vi "Voltage_vs_field.vi"() -> ()   [LabVIEW 2015]
uses:
  <vilib>/Utility/file.llb/Write To Spreadsheet File (string).vi
panel:
  out "Data Point":i32
  out "PS Output (A)":dbl
  in  "Filename Label (optional)":string
  out "Voltage (uV)":dbl
  out "Field (Oe)":dbl
  in  "Power Supply Precision (2-5)":dbl=3.0
  in  "Save Output to:":path=path "C:/VNA-FMR user/Desktop/HV loop"
  in  "Voltmeter Rate (0.1-5)":string="5"
  in  "Gaussmeter Address":string="22"
  in  "Nano Voltmeter Address":string="9"
  in  "Power Supply Address":string="6"
  out "XY Graph":cluster{dbl[], dbl[]}(graph)
  in  "Data Points":dbl=501.0
  in  "Field Range (Oe)":dbl=500.0
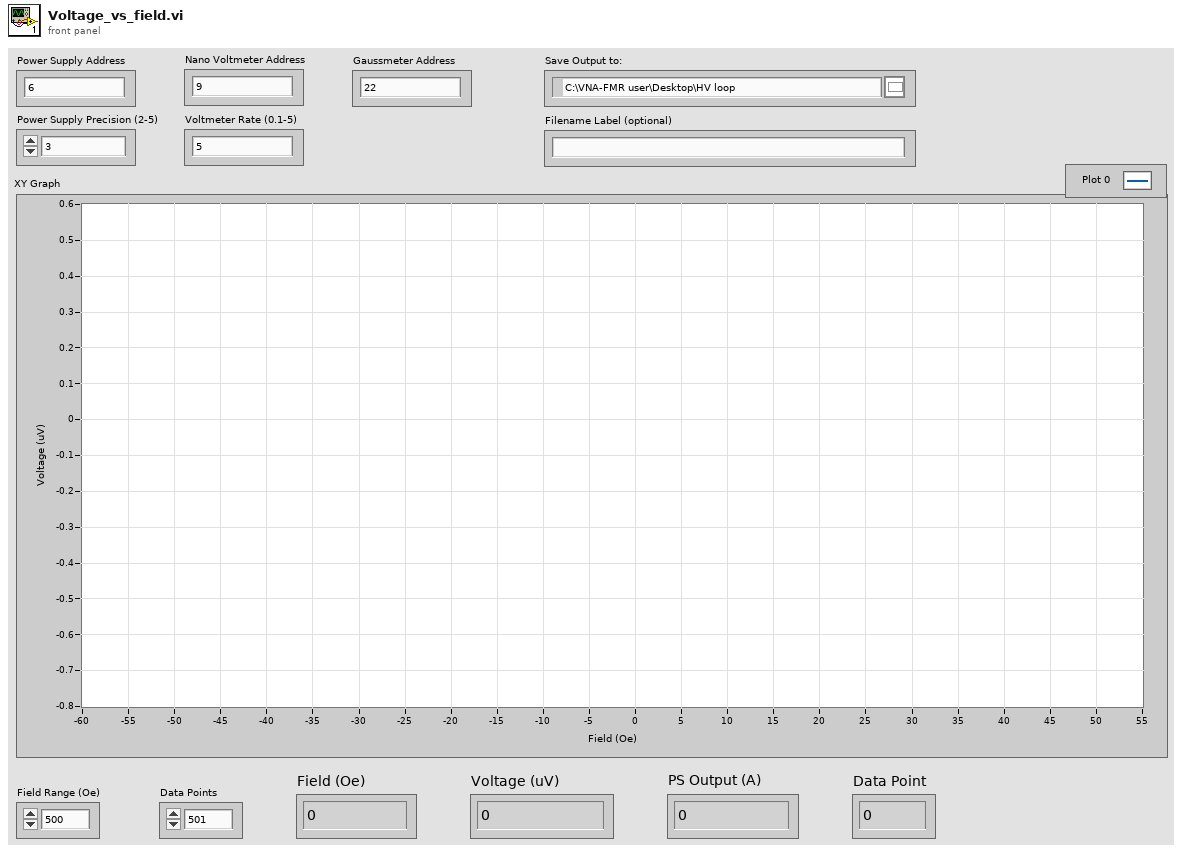
[diagram p1: front panel]
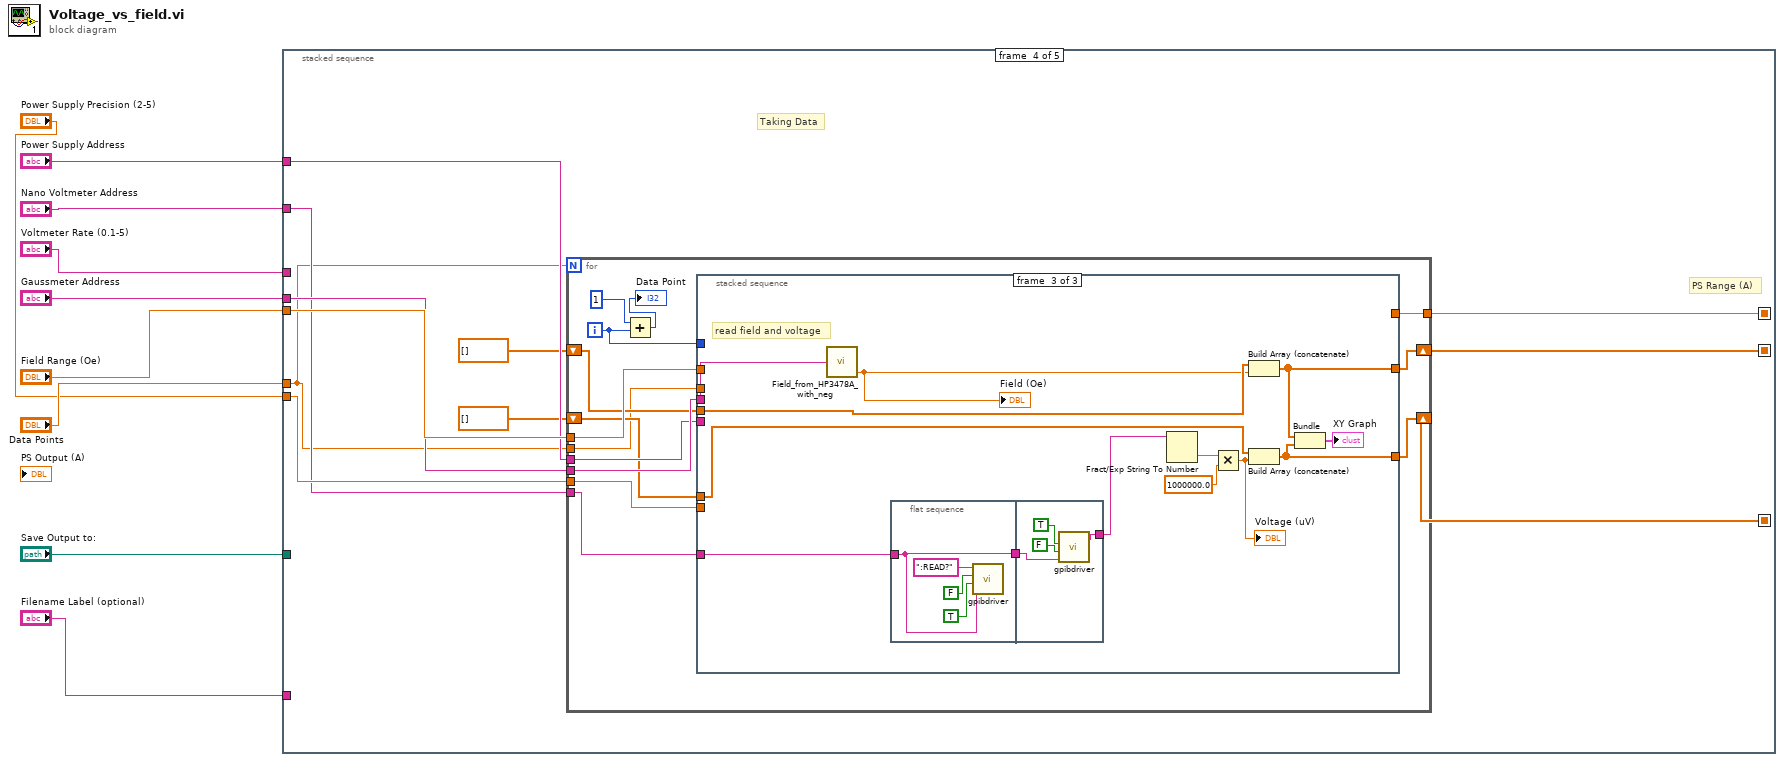
[diagram p0: block diagram]
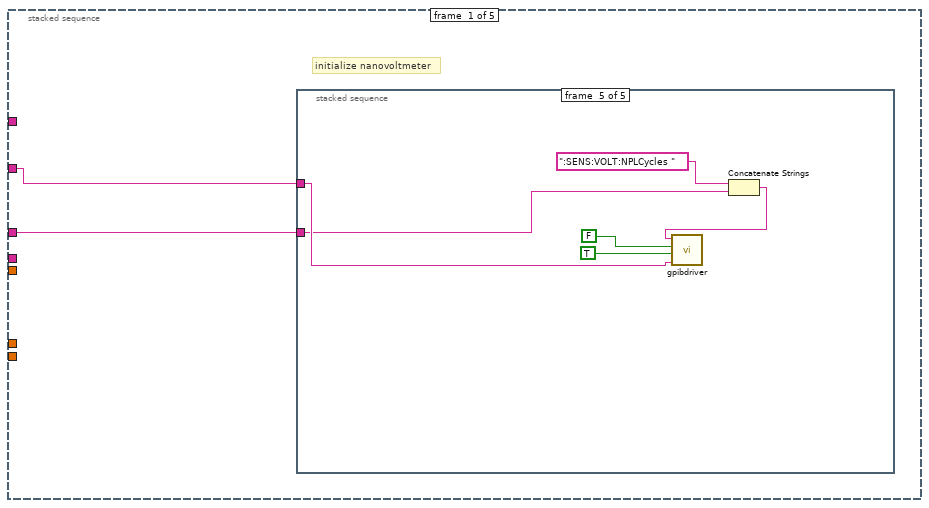
[diagram p2: hidden frame]
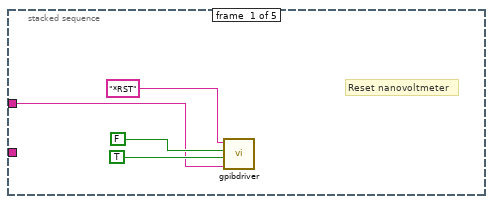
[diagram p3: hidden frame]
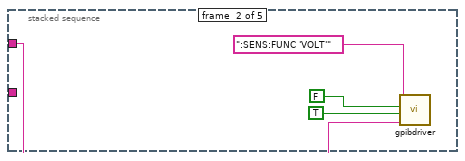
[diagram p4: hidden frame]
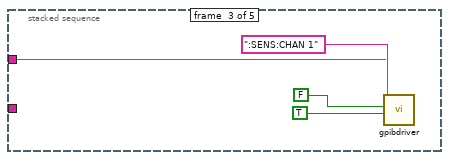
[diagram p5: hidden frame]
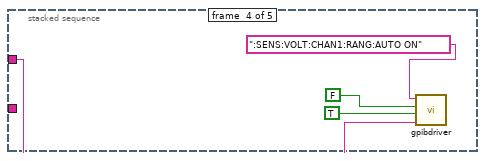
[diagram p6: hidden frame]
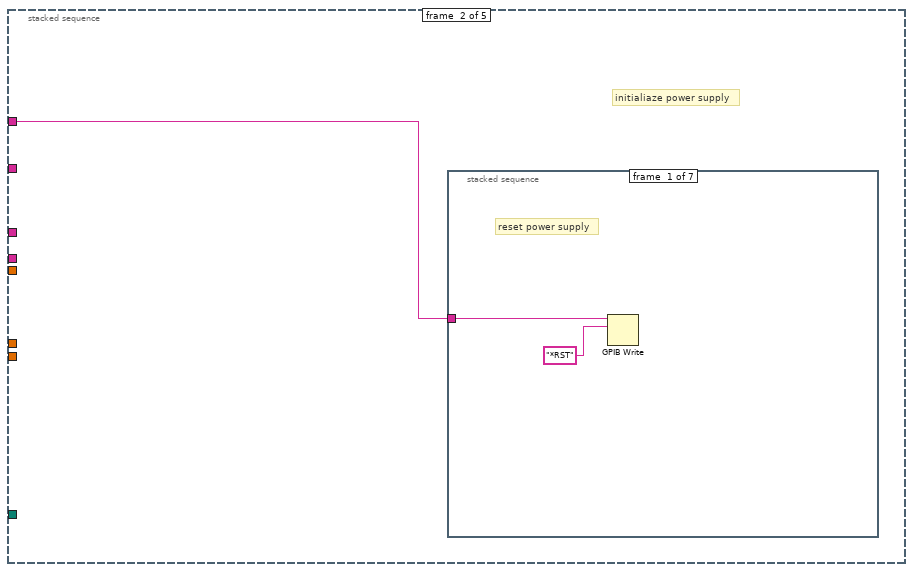
[diagram p7: hidden frame]
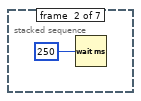
[diagram p8: hidden frame]
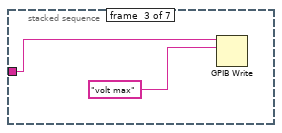
[diagram p9: hidden frame]
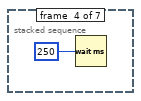
[diagram p10: hidden frame]
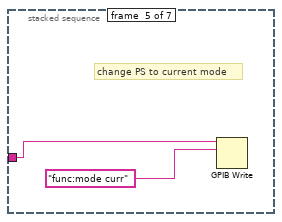
[diagram p11: hidden frame]
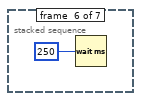
[diagram p12: hidden frame]
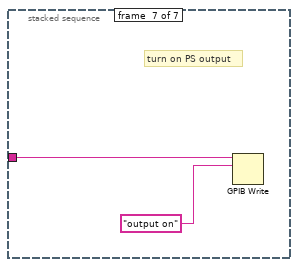
[diagram p13: hidden frame]
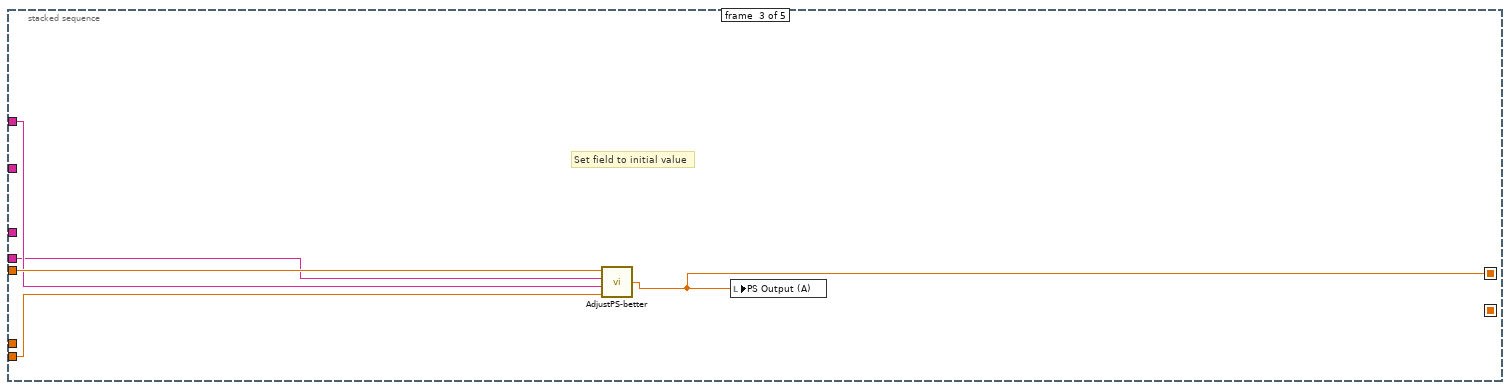
[diagram p14: hidden frame]
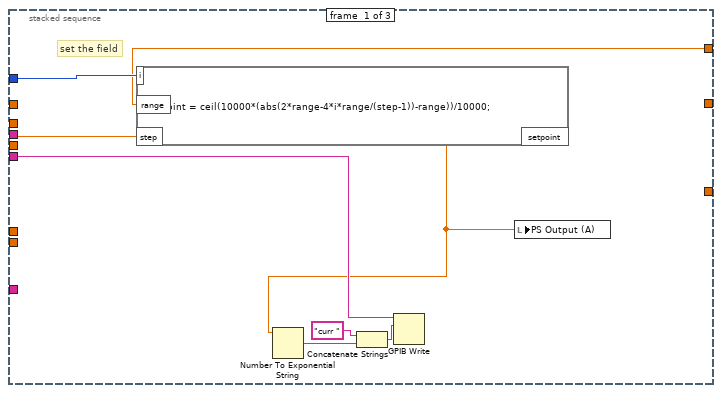
[diagram p15: hidden frame]
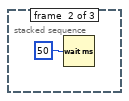
[diagram p16: hidden frame]
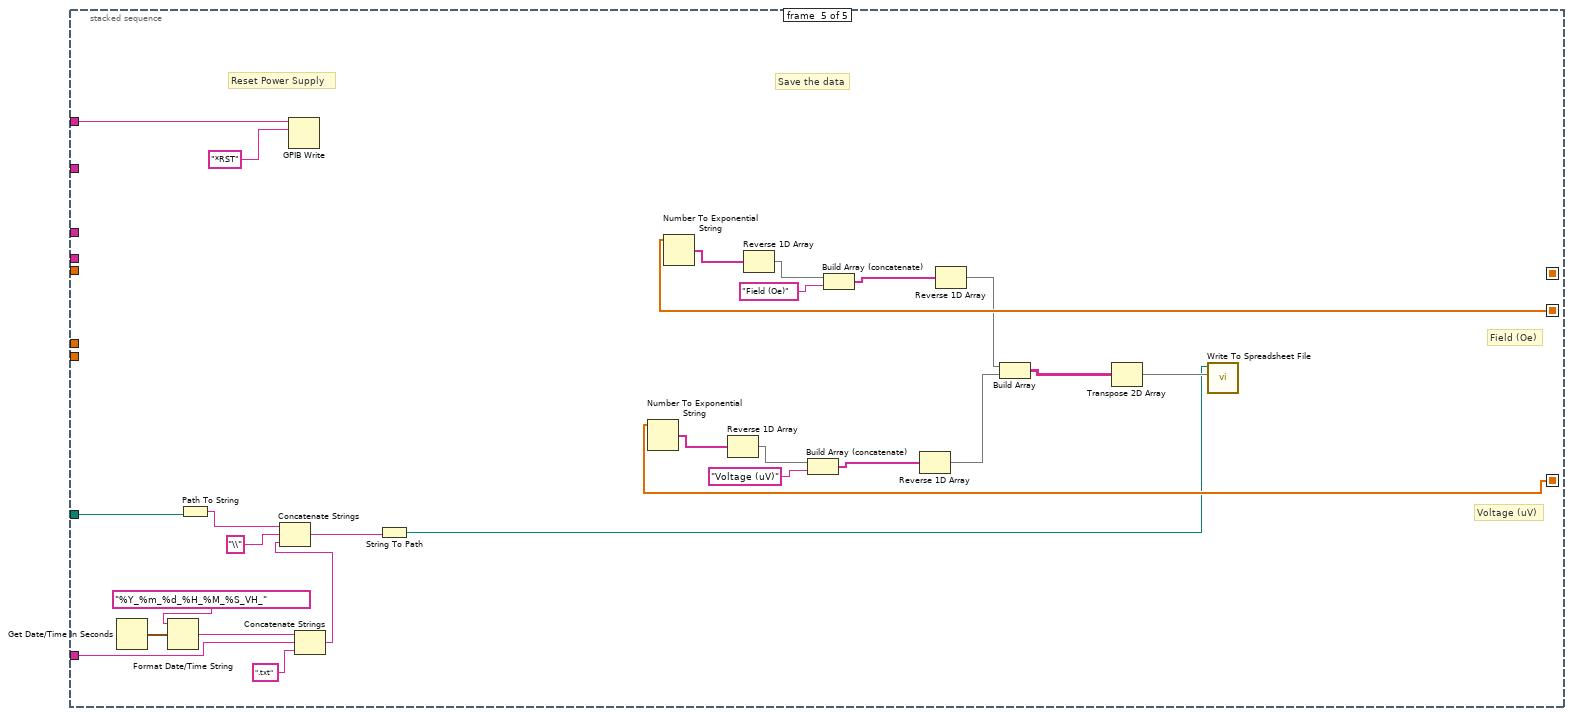
[diagram p17: hidden frame]
diagram:
  n1 = stacked-sequence {
    seq-local: [_ _ _ w54 _] -> [_ _ _ _ w125]
    seq-local: [_ _ _ w53 _] -> [_ _ _ _ w118]
    seq-local: [_ _ w46 _ _] -> [_ _ _ w51 _]
    tunnel: "Nano Voltmeter Address" -> [w11 _ _ w57 _]
    tunnel: "Voltmeter Rate (0.1-5)" -> [w10 _ _ _ _]
    tunnel: "Power Supply Address" -> [_ w34 w49 w59 w132]
    tunnel: "Field Range (Oe)" -> [_ _ w50 w61 _]
    tunnel: "Gaussmeter Address" -> [_ _ w48 w60 _]
    tunnel: "Data Points" -> [_ _ _ w52 _]
    tunnel: "Power Supply Precision (2-5)" -> [_ _ w47 w58 _]
    tunnel: "Save Output to:" -> [_ _ _ _ w116]
    tunnel: "Filename Label (optional)" -> [_ _ _ _ w108]
    frame #0 {
      # "initialize nanovoltmeter"
      n2 = stacked-sequence {
        tunnel: w11 -> [w12 w16 w20 w24 w29]
        tunnel: w10 -> [_ _ _ _ w28]
        frame #0 {
          # "Reset nanovoltmeter"
          n3 = call "gpibdriver.vi"("Characters to Write"="*RST", "Read"=FALSE, "Write"=TRUE ("Write 3"), "GPIB\nAddress"=w12) -> ()  [unwired: 2 in, 1 out]
        }
        frame #1 {
          n4 = call "gpibdriver.vi"("Characters to Write"=":SENS:FUNC 'VOLT'", "Read"=FALSE, "Write"=TRUE ("Write 3"), "GPIB\nAddress"=w16) -> ()  [unwired: 2 in, 1 out]
        }
        frame #2 {
          n5 = call "gpibdriver.vi"("Characters to Write"=":SENS:CHAN 1", "Read"=FALSE, "Write"=TRUE ("Write 3"), "GPIB\nAddress"=w20) -> ()  [unwired: 2 in, 1 out]
        }
        frame #3 {
          n6 = call "gpibdriver.vi"("Characters to Write"=":SENS:VOLT:CHAN1:RANG:AUTO ON", "Read"=FALSE, "Write"=TRUE ("Write 3"), "GPIB\nAddress"=w24) -> ()  [unwired: 2 in, 1 out]
        }
        frame #4 {
          n7 = Concatenate Strings(":SENS:VOLT:NPLCycles " ("Characters to Write"), w28) -> (w33:string)
          n8 = call "gpibdriver.vi"("Characters to Write"=w33, "Read"=FALSE, "Write"=TRUE ("Write 3"), "GPIB\nAddress"=w29) -> ()  [unwired: 2 in, 1 out]
        }
      }
    }
    frame #1 {
      # "initialiaze power supply"
      n9 = stacked-sequence {
        tunnel: w34 -> [w35 _ w39 _ w42 _ w45]
        frame #0 {
          # "reset power supply"
          n10 = GPIB Write(0:w35, 1:"*RST" ("data")) -> ()  [unwired: 3 in, 2 out]
        }
        frame #1 {
          n11 = Wait (ms)(milliseconds to wait=u32 250) -> ()  [unwired: 1 out]
        }
        frame #2 {
          n12 = GPIB Write(0:w39, 1:"volt max" ("data")) -> ()  [unwired: 3 in, 2 out]
        }
        frame #3 {
          n13 = Wait (ms)(milliseconds to wait=u32 250) -> ()  [unwired: 1 out]
        }
        frame #4 {
          # "change PS to current mode"
          n14 = GPIB Write(0:w42, 1:"func:mode curr" ("data")) -> ()  [unwired: 3 in, 2 out]
        }
        frame #5 {
          n15 = Wait (ms)(milliseconds to wait=u32 250) -> ()  [unwired: 1 out]
        }
        frame #6 {
          # "turn on PS output"
          n16 = GPIB Write(0:w45, 1:"output on" ("data")) -> ()  [unwired: 3 in, 2 out]
        }
      }
    }
    frame #2 {
      # "Set field to initial value"
      n17 = call "AdjustPS-better.vi"("Number of steps"=w47, "Power Supply Address"=w49, "Gaussmeter Address"=w48, "Field Set Point (Oe)"=w50) -> ("Set PS to (A)"=w46:dbl)
      n18 = local write "PS Output (A)"(w46) -> ()
    }
    frame #3 {
      # "PS Range (A)"
      # "Taking Data"
      n19 = for {
        N: w52 -> [_]
        tunnel: w61 -> [w75]
        tunnel: w52 -> [w66]
        tunnel: w60 -> [w74]
        tunnel: w59 -> [w73]
        tunnel: w58 -> [w72]
        tunnel: w57 -> [w71]
        shift-right: [w68] -> w54
        shift-left: dbl[] [] -> [w70]
        shift-right: [w67] -> w53
        shift-left: dbl[] [] -> [w69]
        tunnel: w51 -> [w65]
        i -> [w63]
        n20 = Add(x=1, y=w63) -> (x+y=→"Data Point":i32)
        n21 = stacked-sequence {
          tunnel: w75 -> [_ _ _]
          tunnel: w63 -> [w83 _ _]
          tunnel: w66 -> [w82 _ _]
          tunnel: w74 -> [_ _ w97]
          tunnel: w73 -> [w78 _ _]
          tunnel: w72 -> [_ _ _]
          tunnel: w71 -> [_ _ w96]
          tunnel: w70 -> [_ _ w91]
          tunnel: w69 -> [_ _ w89]
          tunnel: [_ _ w86] -> w68
          tunnel: [_ _ w85] -> w67
          tunnel: w65 -> [w77 _ _]
          frame #0 {
            # "set the field"
            n22 = formula code="setpoint = ceil(10000*(abs(2*range-4*i*range/(step-1))-range))/10000;"("i"=w83, "range"=w77, "step"=w82) -> ("setpoint"=w76:dbl)
            n23 = Number To Exponential String(number=w76) -> (E-format string=w81:string)  [unwired: 3 in]
            n24 = Concatenate Strings("curr " ("string"), w81) -> (w79:string)
            n25 = GPIB Write(0:w78, 1:w79) -> ()  [unwired: 3 in, 2 out]
            n26 = local write "PS Output (A)"(w76) -> ()
          }
          frame #1 {
            n27 = Wait (ms)(milliseconds to wait=u32 50) -> ()  [unwired: 1 out]
          }
          frame #2 {
            # "read field and voltage"
            n28 = call "Field_from_HP3478A_with_neg.vi"("GPIB Address"=w97) -> ("Oe"=w90:dbl)  [unwired: 2 out]
            "Field (Oe)" <- w90
            n29 = flat-sequence {
              tunnel: w96 -> [w98]
              tunnel: [w98] -> w95
              tunnel: w95 -> [w103]
              tunnel: [w102] -> w94
              frame #0 {
                n30 = call "gpibdriver.vi"("Characters to Write"=":READ?", "Read"=FALSE, "Write"=TRUE, "GPIB\nAddress"=w98) -> ()  [unwired: 2 in, 1 out]
              }
              frame #1 {
                n31 = call "gpibdriver.vi"("Read"=TRUE, "Write"=FALSE, "GPIB\nAddress"=w103) -> ("Characters Read"=w102:string)  [unwired: 3 in]
              }
            }
            n32 = Fract/Exp String To Number(string=w94) -> (number=w93:dbl)  [unwired: 3 in, 1 out]
            n33 = Multiply(x=w93, y=1000000.0) -> (x*y=w88:dbl)
            "Voltage (uV)" <- w88
            n34 = Build Array (concatenate)(w91, w90) -> (w86:dbl[])
            n35 = Build Array (concatenate)(w89, w88) -> (w85:dbl[])
            n36 = Bundle(w86, w85) -> (→"XY Graph":cluster{dbl[], dbl[]})  [unwired: 1 in]
          }
        }
      }
    }
    frame #4 {
      # "Voltage (uV)"
      # "Field (Oe)"
      # "Save the data"
      # "Reset Power Supply"
      n37 = Get Date/Time In Seconds() -> (seconds since 1Jan1904=w111:timestamp)
      n38 = Format Date/Time String(time format string (%c)="%Y_%m_%d_%H_%M_%S_VH_", seconds (now)=w111) -> (date/time string=w113:string)  [unwired: 1 in]
      n39 = Path To String(path=w116) -> (string=w115:string)
      n40 = GPIB Write(0:w132, 1:"*RST" ("data")) -> ()  [unwired: 3 in, 2 out]
      n41 = Concatenate Strings(w113, w108, ".txt" ("string")) -> (w110:string)
      n42 = Concatenate Strings(w115, "\\" ("string"), w110) -> (w107:string)
      n43 = String To Path(string=w107) -> (path=w106:path)
      n44 = Number To Exponential String(number=w118) -> (E-format string=w120:string[])  [unwired: 3 in]
      n45 = Number To Exponential String(number=w125) -> (E-format string=w126:string[])  [unwired: 3 in]
      n46 = Reverse 1D Array(array=w120) -> (reversed array=w122:string[])
      n47 = Reverse 1D Array(array=w126) -> (reversed array=w128:string[])
      n48 = Build Array (concatenate)(w122, "Voltage (uV)") -> (w121:string[])
      n49 = Build Array (concatenate)(w128, "Field (Oe)") -> (w127:string[])
      n50 = Reverse 1D Array(array=w121) -> (reversed array=w117:string[])
      n51 = Reverse 1D Array(array=w127) -> (reversed array=w123:string[])
      n52 = Build Array(w123, w117) -> (w129:string[][])
      n53 = Transpose 2D Array(2D array=w129) -> (transposed array=w130:string[][])
      n54 = call-poly <vilib>:"Write To Spreadsheet File.vi"("2D data"=w130, "file path (dialog if empty)"=w106) -> ()  [unwired: 6 in, 1 out]
    }
  }
